vi "Get Device Count.vi"(8 "error in (no error)":errorcluster, 11 "RTL-SDR in":refnum<class "RTL-SDR.lvclass">) -> (0 "error out":errorcluster, 2 "Device Count":u32, 3 "RTL-SDR out":refnum<class "RTL-SDR.lvclass">)   [LabVIEW 2015, in "RTL-SDR.lvclass"]
uses:
  RTL-SDR.lvclass
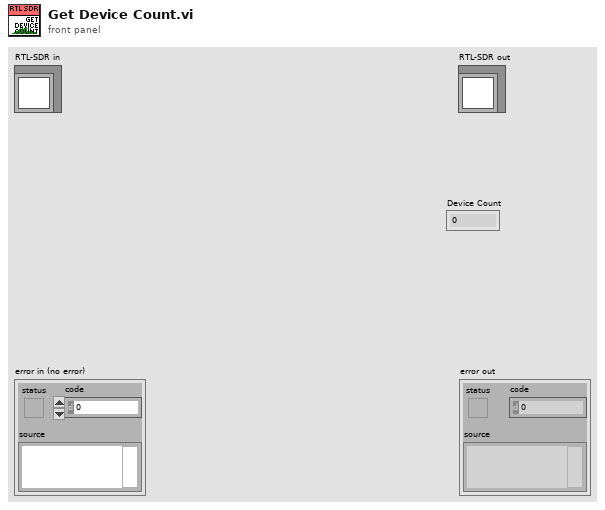
[diagram p1: front panel]
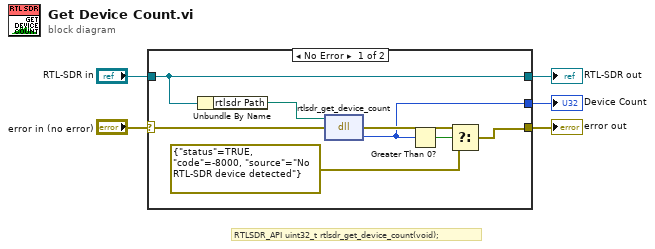
[diagram p0: block diagram]
diagram:
  # "RTLSDR_API uint32_t rtlsdr_get_device_count(void);"
  n1 = case shown="No Error" "error in (no error)" {
    selector: "error in (no error)" -> [w9 w15]
    tunnel: [w10 w15] -> w4
    tunnel: [w13 w14] -> w2
    tunnel: "RTL-SDR in" -> [w13 w14]
    tunnel: [w6 _] -> w1
    frame No Error {
      n2 = Unbundle By Name(w13) -> ("rtlsdr Path"=w7:path)
      n3 = dll-call lib="C:/Users/Ivan/Desktop/D-23-09-24 (RTL-SDR)/Project (Pelleng-SDR)/rtlsdr/dll/rtlsdr.*" fn="rtlsdr_get_device_count"(path in=w7, error in=w9) -> (error out=w8:errorcluster, "return type"=w6:u32)  [unwired: 1 in, 1 out]
      n4 = Greater Than 0?(x=w6) -> (x > 0?=w12:bool)
      n5 = Select(t=w8, s=w12, f=errorcluster {"status"=TRUE, "code"=-8000, "source"="No RTL-SDR device detected"} ("error out")) -> (s? t:f=w10:errorcluster)
    }
    frame Error {
    }
  }
  "error out" <- w4
  "RTL-SDR out" <- w2
  "Device Count" <- w1
